vi "myRIO_BRig_RT_dataExp_FPGA_f_count2ms.vi"() -> (2 "output_FPGA_f_count2ms":i32)   [LabVIEW 2014]
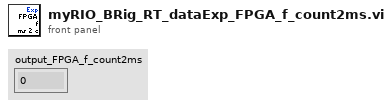
[diagram p1: front panel]
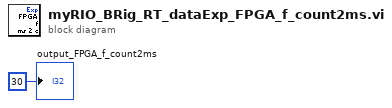
[diagram p0: block diagram]
diagram:
  "output_FPGA_f_count2ms" <- 30 ("output_iBlock")
